vi "Find_SLM_nonbns.vi"(9 "Picture Control":refnum<vi>, 11 "Monitor":i32) -> (1 "Monitor Picture":picture, 2 "Selected Monitor is 1024x768":bool, 3 "Window Rect":i16[](array[numeric]), 4 "Monitor Rect":i16[](array[numeric]), 5 "Sensible Default Monitor":i32)   [LabVIEW 2010]
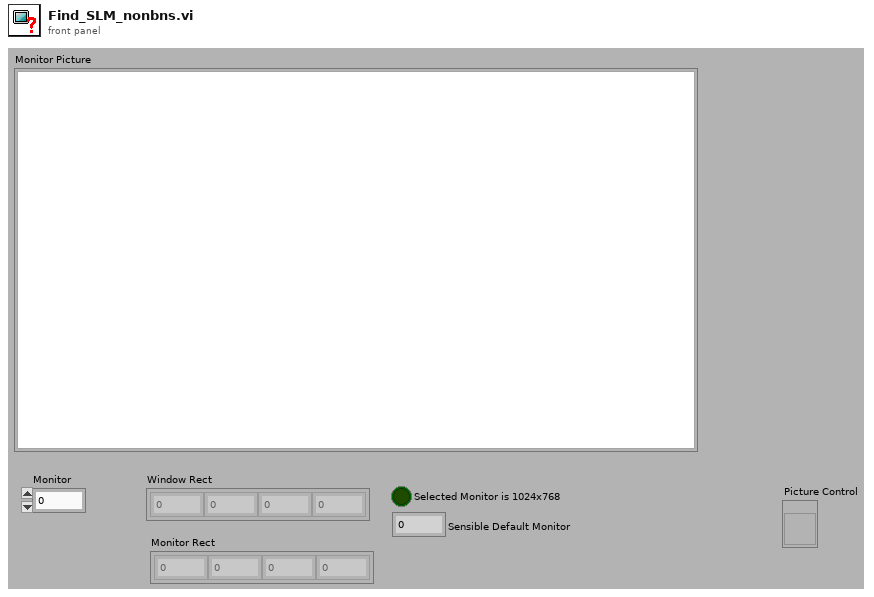
[diagram p1: front panel]
types:
  T1 = typedef "LVAllMonitorsDisplayTypeDef.ctl" = cluster{"Bounds":cluster{"Left":i16, "Top":i16, "Right":i16, "Bottom":i16}, "Depth":i16}[]
  T2 = cluster{"horizontal":enum16{"left", "center", "right"}, "vertical":enum16{"top", "center", "bottom"}}
  T3 = cluster{"Font Name:":string, "Size":i16, "Strikeout?":bool, "Italic?":bool, "Underline?":bool, "Outline?":bool, "Shadow?":bool, "Bold?":bool}
  T4 = enum16{"User-specified Font", "Application Font", "System Font", "Dialog Font"}
  T5 = cluster{"Width":i16, "Style":enum32{"Solid", "Dash", "Dot", "DashDot", "DashDotDot"}}
  T6 = cluster{"Left":i16, "Top":i16, "Right":i16, "Bottom":i16}
  T7 = typedef "LVBoundsTypeDef.ctl" = cluster{"Width":u32, "Height":u32}
  T8 = cluster{"Left":i16, "Top":i16, "Left":i16, "Top":i16}
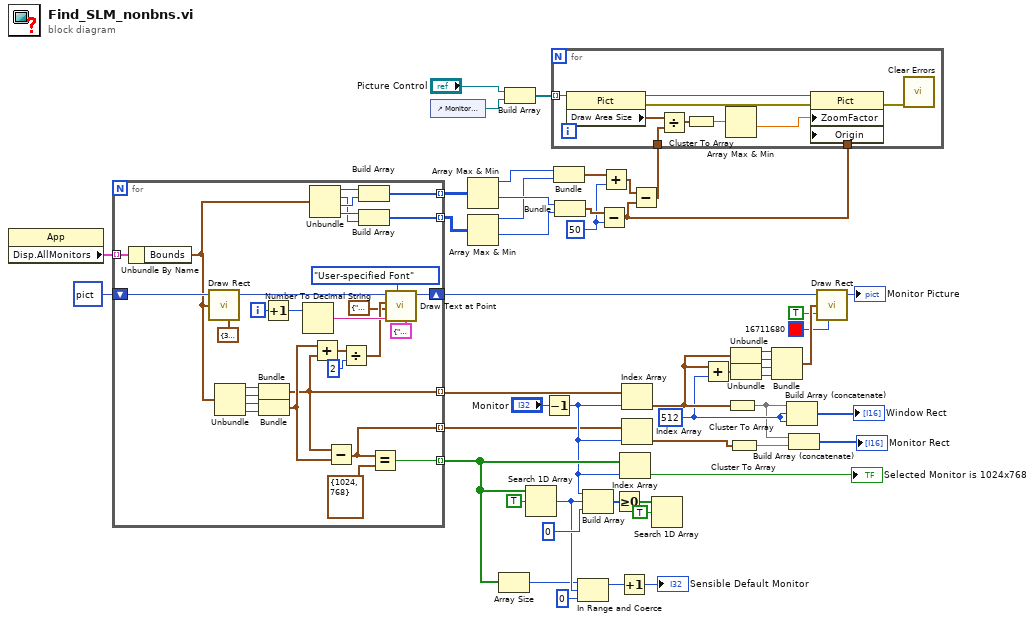
[diagram p0: block diagram]
diagram:
  w23 = i16 512 ("Left")
  w40 = i16 50 ("Left")
  n1 = property class="App"() -> ("Disp.AllMonitors"=w50:T1)  [unwired: 2 in, 2 out]
  n2 = for {
    tunnel: w50 -> [w80] mode=indexing
    shift-right: [w64] -> w36
    shift-left: picture data[5B] ("new picture") -> [w79]
    tunnel: [w73] -> w48 mode=indexing
    tunnel: [w72] -> w47 mode=indexing
    tunnel: [w54] -> w34 mode=indexing
    tunnel: [w53] -> w9 mode=indexing
    tunnel: [w51] -> w5 mode=indexing
    i -> [w62]
    n3 = Unbundle By Name(w80) -> ("Bounds"=w63:T6)
    n4 = call <vilib>:"Draw Rect.vi"("picture"=w79, "rect"=w63, "pen"=T5 {"Width"=3, "Style"=enum."Solid"}) -> ("new picture"=w65:picture)  [unwired: 6 in]
    n5 = Unbundle(w63) -> ("Left"=w71:i16, "Top"=w70:i16, "Right"=w69:i16, "Bottom"=w68:i16)
    n6 = Bundle("Left"=w71, "Top"=w70) -> (w54:cluster{"Left":i16, "Top":i16})  [unwired: 1 in]
    n7 = Bundle("Right"=w69, "Bottom"=w68) -> (w56:cluster{"Right":i16, "Bottom":i16})  [unwired: 1 in]
    n8 = Increment(x=w62) -> (x+1=w52:i32)
    n9 = Number To Decimal String(number=w52) -> (decimal integer string=w61:string)  [unwired: 1 in]
    n10 = Unbundle(w63) -> ("Left"=w77:i16, "Top"=w74:i16, "Right"=w76:i16, "Bottom"=w75:i16)
    n11 = Add(x=w56, y=w54) -> (x+y=w67:cluster{i16, i16})
    n12 = Subtract(x=w54, y=w56) -> (x-y=w51:cluster{i16, i16})
    n13 = Divide(x=w67, y=i16 2 ("Left")) -> (x/y=w58:cluster{dbl, dbl})
    n14 = Build Array(w77, w76) -> (w73:i16[])
    n15 = Build Array(w75, w74) -> (w72:i16[])
    n16 = Equal?(x=w51, y=cluster{i16, i16} {1024, 768}) -> (x = y?=w53:bool)
    n17 = call <vilib>:"Draw Text at Point.vi"("[user-specified font]"=T3 {"Font Name:"="Arial", "Size"=400, "Strikeout?"=FALSE, "Italic?"=FALSE, "Underline?"=FALSE, "Outline?"=FALSE, "Shadow?"=FALSE, "Bold?"=TRUE}, "desired font(Application)"=T4."User-specified Font", "text"=w61, "alignment(left, top)"=T2 {"horizontal"=enum."center", "vertical"=enum."center"}, "origin"=w58, "picture"=w65) -> ("new picture"=w64:picture)  [unwired: 4 in, 1 out]
  }
  n18 = control-ref of="Monitor Picture"() -> (w14:refnum<vi>)
  n19 = Array Max & Min(array=w48) -> (max value=w43:i16, min value=w46:i16)  [unwired: 2 out]
  n20 = Array Max & Min(array=w47) -> (max value=w42:i16, min value=w45:i16)  [unwired: 2 out]
  n21 = Array Size(array=w9) -> (size(s)=w10:i32)
  n22 = Build Array("Picture Control", w14) -> (w13:refnum<vi>[])
  n23 = Search 1D Array(1D array=w9, element=TRUE) -> (index of element=w12:i32)  [unwired: 1 in]
  n24 = Decrement(x="Monitor") -> (x-1=w6:i32)
  n25 = Bundle(w43, w42) -> (w41:cluster{i16, i16})  [unwired: 1 in]
  n26 = Bundle(w46, w45) -> (w44:cluster{i16, i16})  [unwired: 1 in]
  n27 = In Range and Coerce(upper limit=w10, x=w12, lower limit=0) -> (coerced(x)=w8:i32)  [unwired: 1 out]
  n28 = Build Array(w6, w12, 0 ("index of element")) -> (w31:i32[])
  n29 = Subtract(x=w44, y=w40) -> (x-y=w37:cluster{i16, i16})
  n30 = Add(x=w41, y=w40) -> (x+y=w39:cluster{i16, i16})
  n31 = Greater Or Equal To 0?(x=w31) -> (x >= 0?=w29:bool[])
  n32 = Increment(x=w8) -> (x+1=→"Sensible Default Monitor":i32)
  n33 = Index Array(array=w9, index=w6) -> (element=→"Selected Monitor is 1024x768":bool)
  n34 = Index Array(array=w34, index=w6) -> (element=w24:cluster{"Left":i16, "Top":i16})
  n35 = Index Array(array=w5, index=w6) -> (element=w2:cluster{i16, i16})
  n36 = Subtract(x=w39, y=w37) -> (x-y=w38:cluster{i16, i16})
  n37 = for {
    tunnel: w38 -> [w90]
    tunnel: w37 -> [w85]
    tunnel: w13 -> [w81] mode=indexing
    n38 = property on="Property Node" class="Pict"(reference=w81) -> (reference out=w84:refnum<vi>, error out=w83:errorcluster, "Draw Area Size"=w89:T7)  [unwired: 1 in]
    n39 = Divide(x=w89, y=w90) -> (x/y=w88:cluster{dbl, dbl})
    n40 = Cluster To Array(cluster=w88) -> (array=w87:dbl[])
    n41 = Array Max & Min(array=w87) -> (min value=w86:dbl)  [unwired: 3 out]
    n42 = property on="Property Node" class="Pict"(reference=w84, error in=w83, "ZoomFactor"=w86, "Origin"=w85) -> (error out=w82:errorcluster)  [unwired: 1 out]
    n43 = call <vilib>:"Clear Errors.vi"("error in (no error)"=w82) -> ()  [unwired: 6 in, 1 out]
  }
  n44 = Search 1D Array(1D array=w29, element=TRUE) -> ()  [unwired: 1 in, 1 out]
  n45 = Add(x=w24, y=w23) -> (x+y=w25:cluster{"Left":i16, "Top":i16})
  n46 = Cluster To Array(cluster=w24) -> (array=w4:i16[])
  n47 = Cluster To Array(cluster=w2) -> (array=w3:i16[])
  n48 = Unbundle(w24) -> ("Left"=w22:i16, "Top"=w21:i16)
  n49 = Unbundle(w25) -> ("Left"=w20:i16, "Top"=w19:i16)
  n50 = Bundle("Left"=w22, "Top"=w21, "Left"=w20, "Top"=w19) -> (w18:T8)  [unwired: 1 in]
  n51 = Build Array (concatenate)(w4, w23, w23) -> (→"Window Rect":i16[])
  n52 = Build Array (concatenate)(w4, w3) -> (→"Monitor Rect":i16[])
  n53 = call <vilib>:"Draw Rect.vi"("picture"=w36, "rect"=w18, "fill?(F)"=TRUE, "color(black)"=u32 16711680) -> ("new picture"=→"Monitor Picture":picture)  [unwired: 5 in]
